vi "main test.vi"() -> ()   [LabVIEW 2023, in "Thermotron 8800.lvlib"]
uses:
  Thermotron 8800.lvlib
  Private/AuxSelection.ctl
  Private/ActiveChannels.ctl
  Private/Live Aux Number.ctl
  Private/group.ctl
  Private/control module number.ctl
  Private/AnalogInputChannelNumber.ctl
  Private/ThermAlarmNumberBase0.ctl
  Private/get set.ctl
  Private/AnalogInputChannelNumber 1-4.ctl
  Private/Enabled Off On.ctl
  Private/Power Recovery Mode.ctl
  Private/OptionWordSelection.ctl
  Private/ThermAlarmNumber.ctl
  Private/Celcius or Fahrenheit.ctl
  Private/reset.ctl
  <vilib>/NI/Progress Bar/Controls/Update Bar Actions.ctl
panel:
  in  "Input parms":T1={"Controlled stop mode (1=enable; 0=disable)"=1, "Controlled stop set point (0 - 50 deg C)"=30, "Controlled stop purge time (0-3600 seconds)"=10, "Controlled stop deviation (0 - 999.9 deg C)"=5.2, "Controlled stop control mode (1=on; 0=off)"=1}
  out "Software version":string
  out "Temperature scale text":string
  out "Temperature scale\n(0=Celcius; 1=Fahrenheit)":u8
  out "Temperature scale":string
  out "Temperature scale result":string
  out "Time left string 3":string
  out "Time left string 2":string
  out "seconds":i32
  out "minutes":i32
  out "hours":i32
  out "Time left cluster":T2
  out "Time left string 4":string
  out "Time left string 1":string
  out "Throttle reading":i8 format="%0.1f"
  out "Throttle reading string":string
  out "ThermAlarm temperature":i32
  out "ThermAlarm temperature string":string
  out "ThermAlarm analog input value":i32
  out "ThermAlarm analog input value string":string
  out "Reset watchdog timer result":string
  out "Manual ramp setting":sgl
  out "Manual ramp setting string":string
  out "Manual ramp setting status":string
  out "Monitor channel value":sgl
  out "Monitor Channel Value String":string
  out "Operating mode binary":string
  out "Operating mode":u8
  out "Operating mode string":string
  out "Service request event mask binary":string
  out "Service request event mask":i32
  out "Controlled stop parms response":string
  out "Controlled stop parms response from set":string
  out "Number of loops string":string
  out "Number of loops":i32
  out "Next interval":i32
  out "Option response get":string
  out "Option response set":string
  out "High process alarm limit":string
  out "Low process alarm limit":string
  out "Parm response 2":string
  out "Parm response":string
  out "Parameter values response":string
  out "Currently loaded program name response":string
  out "Parameter group":string
  out "Parameter group response":string
  out "8800 program":string
  out "8800 response":string
  out "Program time":string
  out "Program time remaining":string
  out "Process Variable":string
  out "Power fail recovery response":string
  out "Power fail recovery set response":string
  out "Refrigeration system status binary string":string
  out "Refrigeration system status":i32
  out "Refrigeration system status string":string
  out "Refrig system pressures":string
  out "Resume result":string
  out "Real time clock":string
  out "Real time clock set result":string
  out "Stop code":string
  out "reset screen response":string
  out "Chamber serial number":string
  out "Setpoint":dbl format="%.1f"
  out "Setpoint status":string
  out "Service request event mask status":string
  out "Service request event mask string":string
  out "Service request binary string":string
  out "Service request status":i32
  out "Service request status string":string
  out "Service request interval":string
  out "Service request interval status":string
  out "Access level response set":string
  out "Access level response get":string
  out "Loops left?":string
  out "Loops left status":string
  out "Light Status from Set":string
  out "Light Status from Get":string
  out "Enabled? (0=disabled, 1=enabled) 2":i32
  out "Live Aux State (0=off, 1=on) 2":i32
  out "Enabled? (0=disabled, 1=enabled)":i32
  out "Live Aux State (0=off, 1=on)":i32
  in  "State (o=off, 1=on)":i8=1 min=0 max=1 step=1
  in  "Live Aux Number (1-8)":T3=2 min=1 max=8
  out "Language Mode Integer":i32
  out "Language Mode string":string
  out "Current interval initial value":sgl
  out "Current interval initial value string":string
  out "Interval Time":string
  out "analog input channel available?":i32
  in  "Aux Cluster 2":T5={"Group 1 Aux box input"=[2, 4, 5], "Group 2 Aux box input"=[5, 7], "Group 1 Aux code input"=0, "Group 2 Aux code input"=0, "Aux selector box"=TRUE} {"Group 2 Aux code input" min=0 max=255 step=1; "Group 1 Aux code input" min=0 max=255 step=1}
  in  "Interval Parameters Cluster 2":T6={"Final Value 1"=33.2, "Final Value 2"=43.7, "Final Value 3"=0.0, "Final Value 4"=0.0, "Deviation 1"=4.0, "Deviation 2"=5.0, "Deviation 3"=0.0, "Deviation 4"=0.0, "hours"=3, "minutes"=6, "seconds"=7, "Parameter Group"=3, "Number Of Loops"=4, "Next Interval"=1} {"Next Interval" min=0 max=300 step=1; "Number Of Loops" min=0 max=9999 step=1; "Parameter Group" min=1 max=4 step=1; "seconds" min=0 max=99 step=1; "minutes" min=0 max=99 step=1; "hours" min=0 max=99 step=1}
  in  "Interval Parameters Cluster 1":T6={"Final Value 1"=31.2, "Final Value 2"=41.7, "Final Value 3"=0.0, "Final Value 4"=0.0, "Deviation 1"=3.3, "Deviation 2"=4.4, "Deviation 3"=0.0, "Deviation 4"=0.0, "hours"=2, "minutes"=4, "seconds"=5, "Parameter Group"=2, "Number Of Loops"=0, "Next Interval"=2} {"Next Interval" min=0 max=300 step=1; "Number Of Loops" min=0 max=9999 step=1; "Parameter Group" min=1 max=4 step=1; "seconds" min=0 max=99 step=1; "minutes" min=0 max=99 step=1; "hours" min=0 max=99 step=1}
  out "8800 Get Response INTV2":string
  out "Program number of intervals from set":string
  out "Program get number of intervals":string
  out "8800 Get Response from INTV 0":string
  out "8800 Set Response from INTV 0":string
  in  "Interval Parameters Cluster 0":T6={"Final Value 1"=29.2, "Final Value 2"=39.7, "Final Value 3"=0.0, "Final Value 4"=0.0, "Deviation 1"=1.1, "Deviation 2"=2.2, "Deviation 3"=0.0, "Deviation 4"=0.0, "hours"=1, "minutes"=2, "seconds"=3, "Parameter Group"=1, "Number Of Loops"=0, "Next Interval"=1} {"Next Interval" min=0 max=300 step=1; "Number Of Loops" min=0 max=9999 step=1; "Parameter Group" min=1 max=4 step=1; "seconds" min=0 max=99 step=1; "minutes" min=0 max=99 step=1; "hours" min=0 max=99 step=1}
  in  "Active Channels Cluster":T8={"Active Channels box input"=[1, 2], "Active Channels code input"=7, "Active Channels selector T(box) F(code)"=FALSE} {"Active Channels code input" min=0 max=15 step=1}
  in  "Aux Cluster 1":T5={"Group 1 Aux box input"=[1, 3], "Group 2 Aux box input"=[6, 8], "Group 1 Aux code input"=9, "Group 2 Aux code input"=12, "Aux selector box"=FALSE} {"Group 2 Aux code input" min=0 max=255 step=1; "Group 1 Aux code input" min=0 max=255 step=1}
  out "8800 Get Response from INTV1":string
  out "8800 Set Response from INTV 2":string
  out "8800 Set Response from INTV1":string
  out "Interval Number":i32
  out "Interval Number string":string
  out "Last error code":string
  out "8800 Response Identification scpi":string
  out "8800 Response Identification":string
  out "8800 Response":string
  out "Data Type":string
  out "Reference Data Type":string
  out "Door Status":string
  out "Program Directory":string
  out "Digital Output Status binary extended":string
  out "Digital Output Status extended":i32
  out "Digital Output Status string extended":string
  out "Digital Output Status binary":string
  out "Digital Output Status":i32
  out "Digital Output Status string":string
  out "Digital Input Status binary":string
  out "Digital Input Status":i32
  out "Digital Input Status string":string
  out "set deviation response":string
  out "get deviation response":string
  out "Active channel status":i32
  out "Active channel status string":string
  out "version number of control module":string
  out "Channel on and configured status binary":string
  out "analog therm-alarm settings":string[](array[string])
  out "set result talrm settings":string
  out "Configured Options binary string":string
  out "Configured Options":i32
  out "Configured Options string":string
  out "Name of channel":string
  out "Comm status String Value":string
  out "Comm status Value":i32
  out "Channel on and configured status":string
  out "channel run time":string
  out "channel configuration information":string
  out "ascii units character":string
  out "Alarm status":i32
  out "Aux Decimal Value":i32
  out "Aux String Value":string
  out "Alarm status string":string
  out "ThermAlarm analog input units value":string
  out "Instrument Firmware Revision":string
  out "Instrument Driver Revision":string
  out "error out":errorcluster
  in  "error in (no error)":errorcluster
  in  "VISA resource name":refnum<visa-resource-name>="TCPIP::192.168.2.102::8888::SOCKET"
  # "Select Aux boxes"
  # "Select Aux code"
  # "Select Active Channels boxes"
  # "Select Active Channels code"
  # "Select Aux boxes"
  # "Select Aux code"
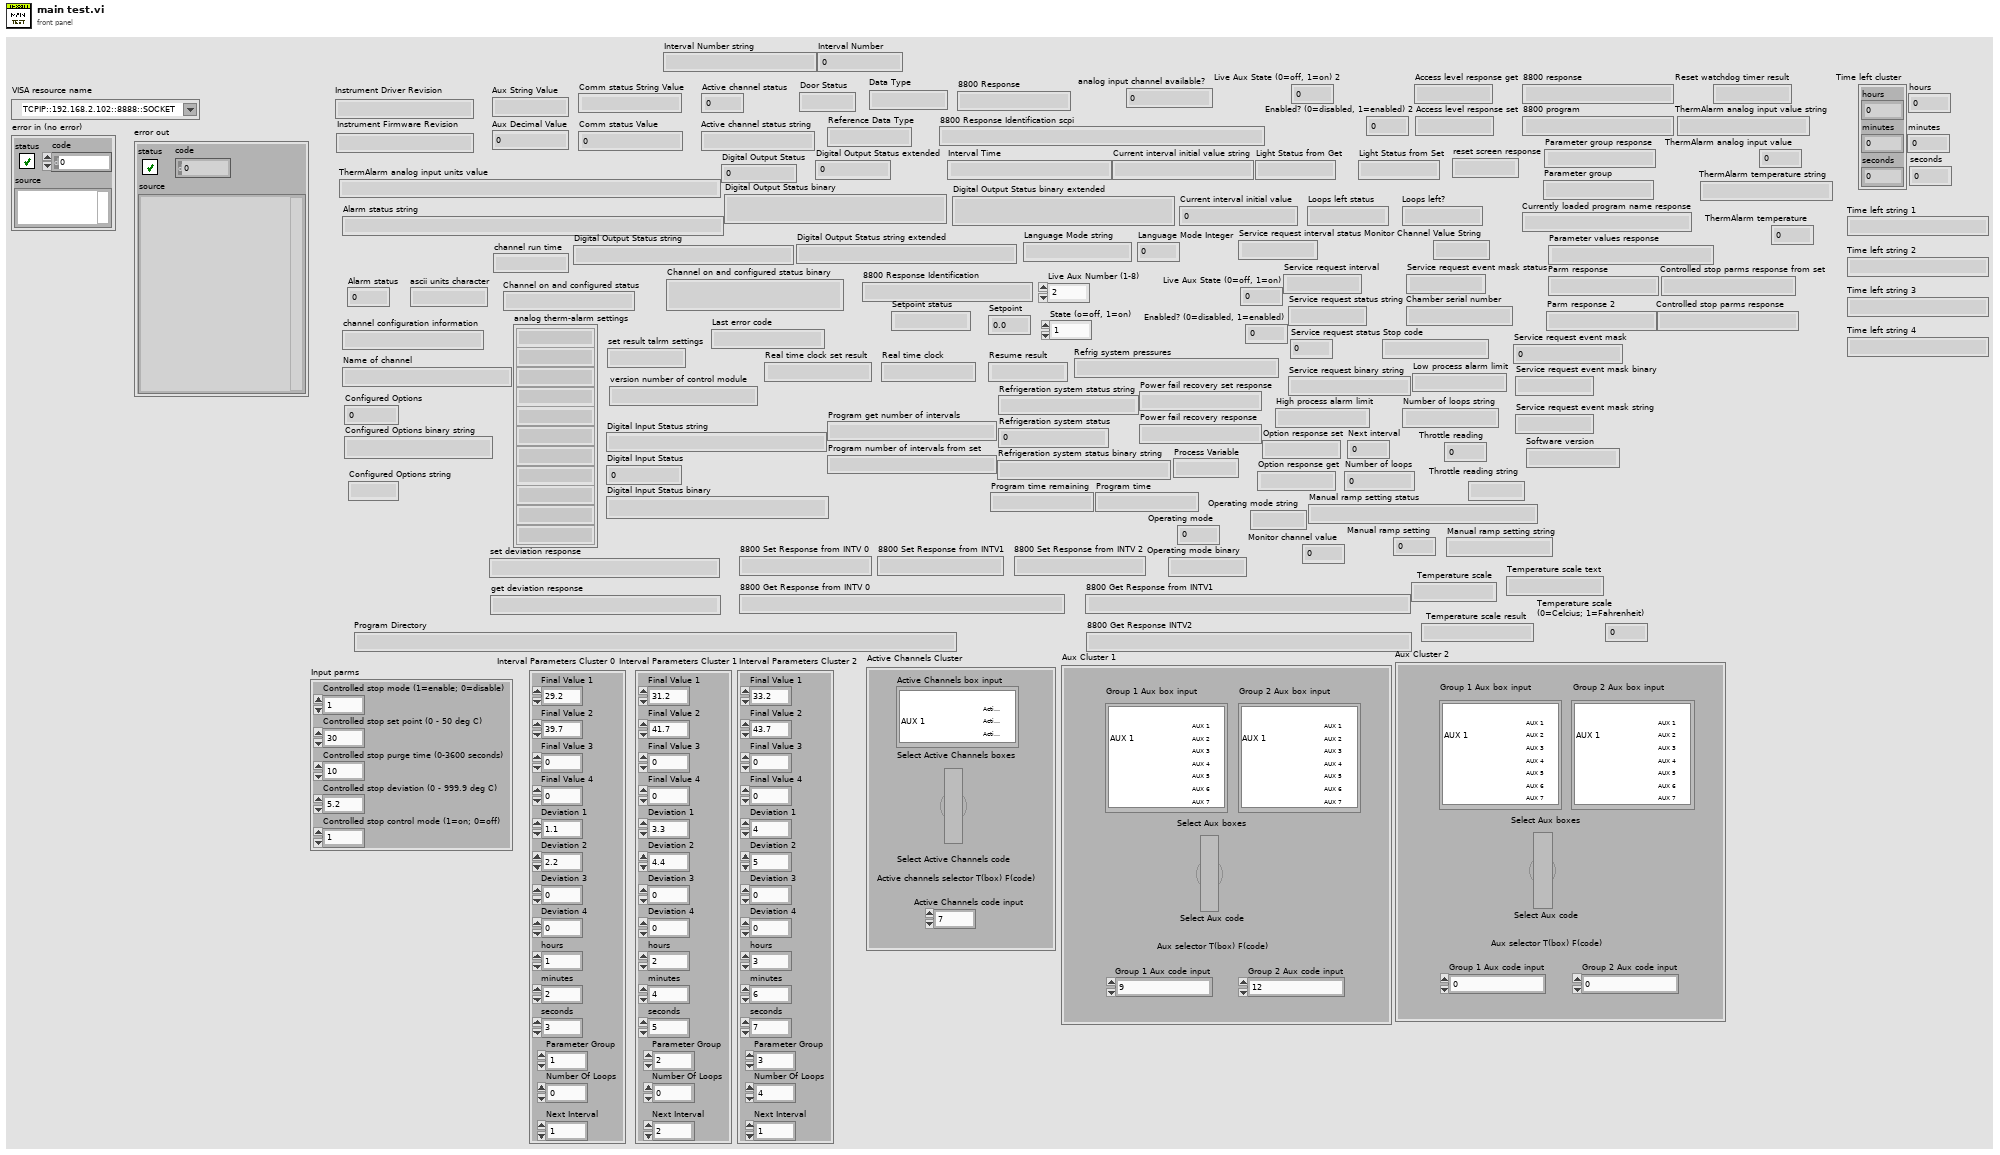
[diagram p1: front panel]
types:
  T1 = cluster{"Controlled stop mode (1=enable; 0=disable)":u8, "Controlled stop set point (0 - 50 deg C)":u8, "Controlled stop purge time (0-3600 seconds)":u16, "Controlled stop deviation (0 - 999.9 deg C)":sgl, "Controlled stop control mode (1=on; 0=off)":u8}
  T2 = cluster{"hours":i32, "minutes":i32, "seconds":i32}
  T3 = typedef "Thermotron 8800.lvlib/Live Aux Number.ctl" = i8
  T4 = typedef "Thermotron 8800.lvlib/AuxSelection.ctl" = i32[]
  T5 = cluster{"Group 1 Aux box input":T4, "Group 2 Aux box input":T4, "Group 1 Aux code input":i32, "Group 2 Aux code input":i32, "Aux selector box":bool}
  T6 = cluster{"Final Value 1":sgl, "Final Value 2":sgl, "Final Value 3":sgl, "Final Value 4":sgl, "Deviation 1":sgl, "Deviation 2":sgl, "Deviation 3":sgl, "Deviation 4":sgl, "hours":i8, "minutes":i8, "seconds":i8, "Parameter Group":i8, "Number Of Loops":i16, "Next Interval":i16}
  T7 = typedef "Thermotron 8800.lvlib/ActiveChannels.ctl" = i32[]
  T8 = cluster{"Active Channels box input":T7, "Active Channels code input":i32, "Active Channels selector T(box) F(code)":bool}
  T9 = cluster{"Hours\n(0-99)":u8, "Minutes\n(0-5999)":u16, "Seconds\n(0-359999)":u32}
  T10 = typedef "Thermotron 8800.lvlib/reset.ctl" = u16
  T11 = cluster{"warn":i32, "mute":i32, "High Limit":i32, "Low Limit":i32, "delay":i32, "reset":T10}
  T12 = cluster{"Month":string, "Day":string, "Hour":string, "Minute":string}
  T13 = typedef "Thermotron 8800.lvlib/Celcius or Fahrenheit.ctl" = u8
  T14 = typedef "Thermotron 8800.lvlib/get set.ctl" = enum16{"get", "set"}
  T15 = typedef "Thermotron 8800.lvlib/AnalogInputChannelNumber.ctl" = u16
  T16 = typedef "Thermotron 8800.lvlib/ThermAlarmNumber.ctl" = u16
  T17 = typedef "Thermotron 8800.lvlib/AnalogInputChannelNumber 1-4.ctl" = u16
  T18 = typedef "Thermotron 8800.lvlib/OptionWordSelection.ctl" = u16
  T19 = cluster{"Heat Gain":sgl, "Heat IT":u16, "Heat Off":sgl, "Cool Off":sgl, "Cool Gain":sgl, "Cool IT":u16}
  T20 = cluster{"Heat PB":sgl, "Heat IT":u16, "Heat TL":sgl, "Cool TL":sgl, "Cool PB":sgl, "Cool IT":u16}
  T21 = typedef "Thermotron 8800.lvlib/Power Recovery Mode.ctl" = u8
  T22 = typedef "Thermotron 8800.lvlib/Enabled Off On.ctl" = u8
  T23 = typedef "Thermotron 8800.lvlib/control module number.ctl" = u16
  T24 = typedef "Thermotron 8800.lvlib/ThermAlarmNumberBase0.ctl" = u16
  T25 = typedef "Thermotron 8800.lvlib/group.ctl" = enum16{"Group1", "Group2"}
  T26 = typedef "Progress Bar.lvlib/Update Bar Actions.ctl" = enum16{"Add To Existing", "Set to Value"}
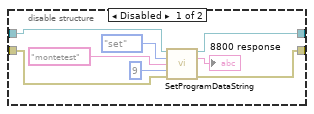
[diagram p2: hidden frame]
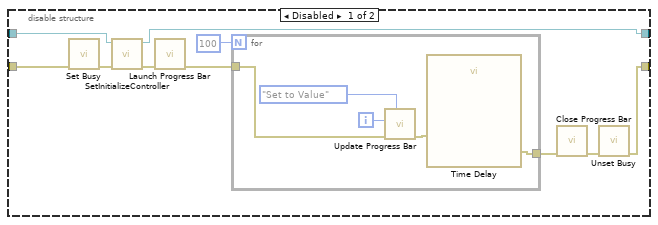
[diagram p3: hidden frame]
diagram:
  w17 = T13 0 items=["Celcius", "Fahrenheit"] ("Temperature scale")
  w24 = get_set."get" ("get/set")
  w43 = get_set."set" ("get/set")
  w50 = T15 2 items=["Channel 1"=1, "Channel 2"=2, "Channel 3"=3, "Channel 4"=4, "Channel 5"=5, "Channel 6"=6, "Channel 7"=7, "Channel 8"=8] ("Channel Number (1-8)")
  w55 = T16 1 items=["ThermAlarm 1"=1, "ThermAlarm 2"=2, "ThermAlarm 3"=3, "ThermAlarm 4"=4] ("ThermAlarm number")
  w71 = T17 1 items=["Channel 1"=1, "Channel 2"=2, "Channel 3"=3, "Channel 4"=4] ("Channel Number (1-4)")
  w106 = T18 8 items=["Product temperature control"=1, "Humidity system"=2, "Low humidity system"=4, "GSoak"=8, "Purge"=16, "Cascade refrigeration"=32, "Power Save mode"=64, "Single-stage refrig."=128, "Altitude"=512, "Mechanical boost"=1024, "Product dewpoint control"=32768] ("Option (may be added for multiple)")
  w116 = T17 1 items=["Channel 1"=1, "Channel 2"=2, "Channel 3"=3, "Channel 4"=4] ("Channel Number (1-4)")
  w141 = "%.1f" ("format string")
  w148 = string[] [","] ("delimiters (\\s,\\t,\\r,\\n)")
  w133 = u8 1 ("Parameter group number (1-4)")
  w134 = T17 1 items=["Channel 1"=1, "Channel 2"=2, "Channel 3"=3, "Channel 4"=4] ("Control channel number (1-4)")
  w135 = get_set."set" ("get/set")
  w195 = T21 2 items=["stop", "hold", "run", "restart"] ("Power Recovery Mode")
  w199 = T22 1 items=["Off", "On"] ("Enabled?")
  w209 = T17 1 items=["Channel 1"=1, "Channel 2"=2, "Channel 3"=3, "Channel 4"=4] ("Refrigeration system number (1-4)")
  w211 = T17 1 items=["Channel 1"=1, "Channel 2"=2, "Channel 3"=3, "Channel 4"=4] ("Refrig system number (1-4)")
  w235 = T17 1 items=["Channel 1"=1, "Channel 2"=2, "Channel 3"=3, "Channel 4"=4] ("Channel Number (1-4)")
  w290 = get_set."get" ("get/set")
  w291 = get_set."set" ("get/set")
  w319 = T17 1 items=["Channel 1"=1, "Channel 2"=2, "Channel 3"=3, "Channel 4"=4] ("Channel Number (1-4)")
  w326 = T16 1 items=["ThermAlarm 1"=1, "ThermAlarm 2"=2, "ThermAlarm 3"=3, "ThermAlarm 4"=4] ("ThermAlarm number")
  w354 = "test" ("8800 Program Name")
  w365 = i16 0 ("Interval Number")
  w338 = i16 2 ("Interval Number")
  w360 = i16 1 ("Interval Number")
  w337 = get_set."get" ("get/set")
  w366 = get_set."set" ("get/set")
  w370 = u16 32 items=["Product temperature control"=1, "Humidity system"=2, "Low humidity system"=4, "GSoak"=8, "Purge"=16, "Cascade refrigeration"=32, "Power Save mode"=64, "Single-stage refrigeration"=128, "Altitude"=512, "Mechanical boost"=1024, "Product dew point control"=32768] ("Options")
  w333 = u16 32 items=["Product temperature control"=1, "Humidity system"=2, "Low humidity system"=4, "GSoak"=8, "Purge"=16, "Cascade refrigeration"=32, "Power Save mode"=64, "Single-stage refrigeration"=128, "Altitude"=512, "Mechanical boost"=1024, "Product dew point control"=32768] ("Options")
  w369 = u16 2 items=["Product temperature control"=1, "Humidity system"=2, "Low humidity system"=4, "GSoak"=8, "Purge"=16, "Cascade refrigeration"=32, "Power Save mode"=64, "Single-stage refrigeration"=128, "Altitude"=512, "Mechanical boost"=1024, "Product dew point control"=32768] ("Options")
  w332 = u16 1024 items=["Product temperature control"=1, "Humidity system"=2, "Low humidity system"=4, "GSoak"=8, "Purge"=16, "Cascade refrigeration"=32, "Power Save mode"=64, "Single-stage refrigeration"=128, "Altitude"=512, "Mechanical boost"=1024, "Product dew point control"=32768] ("Options")
  w331 = u16 2 items=["Product temperature control"=1, "Humidity system"=2, "Low humidity system"=4, "GSoak"=8, "Purge"=16, "Cascade refrigeration"=32, "Power Save mode"=64, "Single-stage refrigeration"=128, "Altitude"=512, "Mechanical boost"=1024, "Product dew point control"=32768] ("Options")
  w393 = T17 1 items=["Channel 1"=1, "Channel 2"=2, "Channel 3"=3, "Channel 4"=4] ("Channel Number (1-4)")
  w417 = T23 2 items=["control module 1"=1, "control module 2"=2, "control module 3"=3, "control module 4"=4] ("control module number")
  w430 = T17 1 items=["Channel 1"=1, "Channel 2"=2, "Channel 3"=3, "Channel 4"=4] ("Channel Number (1-4)")
  w442 = T24 0 items=["ThermAlarm 1", "ThermAlarm 2", "ThermAlarm 3", "ThermAlarm 4"] ("ThermAlarm number")
  w446 = T15 1 items=["Channel 1"=1, "Channel 2"=2, "Channel 3"=3, "Channel 4"=4, "Channel 5"=5, "Channel 6"=6, "Channel 7"=7, "Channel 8"=8] ("Channel Number")
  w444 = T15 2 items=["Channel 1"=1, "Channel 2"=2, "Channel 3"=3, "Channel 4"=4, "Channel 5"=5, "Channel 6"=6, "Channel 7"=7, "Channel 8"=8] ("Channel Number")
  w445 = T15 1 items=["Channel 1"=1, "Channel 2"=2, "Channel 3"=3, "Channel 4"=4, "Channel 5"=5, "Channel 6"=6, "Channel 7"=7, "Channel 8"=8] ("Channel Number")
  w448 = T23 1 items=["control module 1"=1, "control module 2"=2, "control module 3"=3, "control module 4"=4] ("control module number")
  w456 = T16 1 items=["ThermAlarm 1"=1, "ThermAlarm 2"=2, "ThermAlarm 3"=3, "ThermAlarm 4"=4, "ThermAlarm 5"=5, "ThermAlarm 6"=6, "ThermAlarm 7"=7, "ThermAlarm 8"=8] ("ThermAlarm number")
  # "note: SRQM and SRQB are already done"
  # "main test.vi"
  n1 = call "Initialize.vi"("error in (no error)"="error in (no error)", "VISA resource name"="VISA resource name") -> ("error out"=w513:errorcluster, "VISA resource name out"=w512:refnum<visa-resource-name>)  [unwired: 7 in, 1 out]
  n2 = call "Reset.vi"("error in (no error)"=w513, "VISA resource name"=w512) -> ("error out"=w489:errorcluster, "VISA resource name out"=w490:refnum<visa-resource-name>)  [unwired: 8 in]
  n3 = call "Revision Query.vi"("error in (no error)"=w489, "VISA resource name"=w490) -> ("error out"=w508:errorcluster, "Instrument Firmware Revision"=→"Instrument Firmware Revision":string, "Instrument Driver Revision"=→"Instrument Driver Revision":string, "VISA resource name out"=w509:refnum<visa-resource-name>)  [unwired: 6 in]
  n4 = call "GetThermAlarmAnalogInputUnitsValue.vi"("error in"=w508, "ThermAlarm number"=w456, "VISA resource name"=w509) -> ("error out"=w506:errorcluster, "ThermAlarm analog input units value"=→"ThermAlarm analog input units value":string, "VISA resource name out"=w505:refnum<visa-resource-name>)  [unwired: 6 in]
  n5 = call "GetAlarmStatus.vi"("error in"=w506, "Channel Number"=w446, "VISA resource name"=w505) -> ("error out"=w496:errorcluster, "Alarm status"=→"Alarm status":i32, "Alarm status string"=→"Alarm status string":string, "VISA resource name out"=w493:refnum<visa-resource-name>)  [unwired: 5 in]
  n6 = call "GetSetAux.vi"("Aux code input"=173, "error in"=w496, "Group"=group."Group1", "get/set"=get_set."set", "VISA resource name"=w493) -> ("error out"=w495:errorcluster, "VISA resource name out"=w492:refnum<visa-resource-name>)  [unwired: 3 in, 2 out]
  n7 = call "SetRunManual.vi"("error in"=w495, "VISA resource name"=w492) -> ("error out"=w494:errorcluster, "VISA resource name out"=w491:refnum<visa-resource-name>)  [unwired: 7 in, 1 out]
  n8 = call "GetSetAux.vi"("error in"=w494, "Group"=group."Group1", "get/set"=get_set."get", "VISA resource name"=w491) -> ("error out"=w484:errorcluster, "Aux Decimal Value"=→"Aux Decimal Value":i32, "Aux String Value"=→"Aux String Value":string, "VISA resource name out"=w485:refnum<visa-resource-name>)  [unwired: 4 in]
  n9 = call "GetPVUnitsChar.vi"("error in"=w484, "Channel number"=1, "VISA resource name"=w485) -> ("error out"=w482:errorcluster, "ascii units character"=→"ascii units character":string, "VISA resource name out"=w483:refnum<visa-resource-name>)  [unwired: 6 in]
  n10 = call "GetProcessChanConfig.vi"("error in"=w482, "Channel Number"=w445, "VISA resource name"=w483) -> ("error out"=w480:errorcluster, "channel configuration information"=→"channel configuration information":string, "VISA resource name out"=w479:refnum<visa-resource-name>)  [unwired: 6 in]
  n11 = call "GetChanRunTime.vi"("error in"=w480, "Channel Number"=w444, "VISA resource name"=w479) -> ("error out"=w477:errorcluster, "channel run time"=→"channel run time":string, "VISA resource name out"=w476:refnum<visa-resource-name>)  [unwired: 6 in]
  n12 = call "GetChanOnAndConfigStatus.vi"("error in"=w477, "VISA resource name"=w476) -> ("error out"=w472:errorcluster, "Channel on and configured status binary"=→"Channel on and configured status binary":string, "Channel on and configured status string"=→"Channel on and configured status":string, "VISA resource name out"=w470:refnum<visa-resource-name>)  [unwired: 6 in]
  n13 = call "GetSetCommStatus.vi"("error in"=w472, "Coded integer comm status"=1, "get/set"=get_set."set", "VISA resource name"=w470) -> ("error out"=w471:errorcluster, "VISA resource name out"=w469:refnum<visa-resource-name>)  [unwired: 4 in, 2 out]
  n14 = call "GetSetCommStatus.vi"("error in"=w471, "get/set"=get_set."get", "VISA resource name"=w469) -> ("error out"=w466:errorcluster, "Comm status Value"=→"Comm status Value":i32, "Comm status String Value"=→"Comm status String Value":string, "VISA resource name out"=w467:refnum<visa-resource-name>)  [unwired: 5 in]
  n15 = call "GetChanName.vi"("error in"=w466, "Channel number"=1, "VISA resource name"=w467) -> ("error out"=w463:errorcluster, "Name of channel"=→"Name of channel":string, "VISA resource name out"=w462:refnum<visa-resource-name>)  [unwired: 6 in]
  n16 = call "GetConfiguredOptions.vi"("VISA resource name"=w462, "error in"=w463) -> ("VISA resource name out"=w453:refnum<visa-resource-name>, "Configured Options string"=→"Configured Options string":string, "Configured Options"=→"Configured Options":i32, "Configured Options binary string"=→"Configured Options binary string":string, "error out"=w454:errorcluster)  [unwired: 9 in]
  n17 = call "GetSetThermAlarmSettings.vi"("VISA resource name"=w453, "ThermAlarm number"=w442, "get/set"=get_set."set", "Input cluster"=T11 {"warn"=3, "mute"=99, "High Limit"=6, "Low Limit"=2, "delay"=4, "reset"=1}, "error in"=w454) -> ("VISA resource name out"=w452:refnum<visa-resource-name>, "set response"=→"set result talrm settings":string, "error out"=w451:errorcluster)  [unwired: 10 in, 2 out]
  n18 = call "GetSetThermAlarmSettings.vi"("VISA resource name"=w452, "ThermAlarm number"=w442, "get/set"=get_set."get", "error in"=w451) -> ("VISA resource name out"=w449:refnum<visa-resource-name>, "get response"=→"analog therm-alarm settings":string[], "error out"=w450:errorcluster)  [unwired: 11 in, 2 out]
  n19 = call "GetControlModuleVersion.vi"("error in"=w450, "control module number"=w448, "VISA resource name"=w449) -> ("error out"=w440:errorcluster, "version number of control module"=→"version number of control module":string, "VISA resource name out"=w439:refnum<visa-resource-name>)  [unwired: 6 in]
  n20 = call "GetActiveChannelStatus.vi"("error in"=w440, "VISA resource name"=w439) -> ("error out"=w436:errorcluster, "Active channel status"=→"Active channel status":i32, "Active channel status string"=→"Active channel status string":string, "VISA resource name out"=w435:refnum<visa-resource-name>)  [unwired: 6 in]
  n21 = call "GetSetDeviation.vi"("Deviation value"=21.1, "error in"=w436, "Channel Number (1-4)"=w430, "get/set"=get_set."set", "VISA resource name"=w435) -> ("error out"=w434:errorcluster, "Deviation"=→"set deviation response":string, "VISA resource name out"=w433:refnum<visa-resource-name>)  [unwired: 4 in]
  n22 = call "GetSetDeviation.vi"("error in"=w434, "Channel Number (1-4)"=w430, "get/set"=get_set."get", "VISA resource name"=w433) -> ("error out"=w425:errorcluster, "Deviation"=→"get deviation response":string, "VISA resource name out"=w426:refnum<visa-resource-name>)  [unwired: 5 in]
  n23 = call "GetDigitalInputStatus.vi"("VISA resource name"=w426, "error in"=w425) -> ("VISA resource name out"=w418:refnum<visa-resource-name>, "Digital Input Status string"=→"Digital Input Status string":string, "Digital Input Status"=→"Digital Input Status":i32, "Digital Input Status binary"=→"Digital Input Status binary":string, "error out"=w419:errorcluster)  [unwired: 9 in]
  n24 = call "GetDigitalOutputStatus.vi"("VISA resource name"=w418, "error in"=w419) -> ("VISA resource name out"=w421:refnum<visa-resource-name>, "Digital Output Status string"=→"Digital Output Status string":string, "Digital Output Status"=→"Digital Output Status":i32, "Digital Output Status binary"=→"Digital Output Status binary":string, "error out"=w420:errorcluster)  [unwired: 9 in]
  n25 = call "GetDigitalOutputStatus.vi"("VISA resource name"=w421, "control module number"=w417, "Extended?"=TRUE, "error in"=w420) -> ("VISA resource name out"=w406:refnum<visa-resource-name>, "Digital Output Status string"=→"Digital Output Status string extended":string, "Digital Output Status"=→"Digital Output Status extended":i32, "Digital Output Status binary"=→"Digital Output Status binary extended":string, "error out"=w407:errorcluster)  [unwired: 7 in]
  n26 = call "GetProgramDirectory.vi"("error in"=w407, "PathName"="\\", "VISA resource name"=w406) -> ("error out"=w403:errorcluster, "Program Directory"=→"Program Directory":string, "VISA resource name out"=w402:refnum<visa-resource-name>)  [unwired: 6 in]
  n27 = call "GetDoorStatus.vi"("error in"=w403, "VISA resource name"=w402) -> ("error out"=w400:errorcluster, "Door Status"=→"Door Status":string, "VISA resource name out"=w399:refnum<visa-resource-name>)  [unwired: 7 in]
  n28 = call "GetReferenceDataType.vi"("error in"=w400, "Channel Number"=1, "VISA resource name"=w399) -> ("error out"=w397:errorcluster, "Reference Data Type"=→"Reference Data Type":string, "VISA resource name out"=w396:refnum<visa-resource-name>)  [unwired: 6 in]
  n29 = call "GetDataType.vi"("error in (no error)"=w397, "Channel Number (1-4)"=w393, "VISA resource name"=w396) -> ("error out"=w392:errorcluster, "Data Type"=→"Data Type":string, "VISA resource name out"=w391:refnum<visa-resource-name>)  [unwired: 6 in]
  n30 = call "SetHold.vi"("error in"=w392, "VISA resource name"=w391) -> ("error out"=w388:errorcluster, "8800 Response"=→"8800 Response":string, "VISA resource name out"=w389:refnum<visa-resource-name>)  [unwired: 7 in]
  n31 = call "GetDeviceIdentification.vi"("error in"=w388, "VISA resource name"=w389) -> ("error out"=w386:errorcluster, "8800 Response Identification"=→"8800 Response Identification":string, "VISA resource name out"=w385:refnum<visa-resource-name>)  [unwired: 7 in]
  n32 = call "GetDeviceIdentificationSCPI.vi"("error in"=w386, "VISA resource name"=w385) -> ("error out"=w383:errorcluster, "8800 Response Identification"=→"8800 Response Identification scpi":string, "VISA resource name out"=w382:refnum<visa-resource-name>)  [unwired: 7 in]
  n33 = call "GetLastErrorCode.vi"("error in"=w383, "VISA resource name"=w382) -> ("error out"=w376:errorcluster, "Last error code"=→"Last error code":string, "VISA resource name out"=w380:refnum<visa-resource-name>)  [unwired: 7 in]
  n34 = disable-structure shown="Enabled" {
    disable-tunnel: w380 -> [w526 w533]
    disable-tunnel: [w525 w533] -> w379
    disable-tunnel: w376 -> [w524 w532]
    disable-tunnel: [w522 w532] -> w375
    frame Disabled {
      n35 = call <vilib>:"Set Busy.vi"("error in (no error)"=w524) -> ("error out"=w523:errorcluster)  [unwired: 9 in, 1 out]
      n36 = call <instrlib>:"SetInitializeController.vi"("error in"=w523, "VISA resource name"=w526) -> ("error out"=w521:errorcluster, "VISA resource name out"=w525:refnum<visa-resource-name>)  [unwired: 8 in]
      n37 = call <vilib>:"Launch Progress Bar.vi"("error in (no error)"=w521) -> ("error out"=w520:errorcluster)  [unwired: 9 in, 1 out]
      n38 = for {
        N: 100 -> [_]
        tunnel: w520 -> [w531]
        tunnel: [w529] -> w519
        i -> [w527]
        n39 = call <vilib>:"Update Progress Bar.vi"("Action"=Update_Bar_Actions."Set to Value", "error in (no error)"=w531, "Value"=w527) -> ("error out"=w530:errorcluster)  [unwired: 8 in]
        n40 = call "Time Delay"("error in (no error)"=w530) -> ("error out"=w529:errorcluster)  [unwired: 10 in]
      }
      n41 = call <vilib>:"Close Progress Bar.vi"("error in (no error)"=w519) -> ("error out"=w518:errorcluster)  [unwired: 9 in, 1 out]
      n42 = call <vilib>:"Unset Busy.vi"("error in (no error)"=w518) -> ("error out"=w522:errorcluster)  [unwired: 10 in]
    }
    frame Enabled {
    }
  }
  n43 = call "GetIntervalNumber.vi"("error in"=w375, "VISA resource name"=w379) -> ("error out"=w359:errorcluster, "Interval Number"=→"Interval Number":i32, "Interval Number string"=→"Interval Number string":string, "VISA resource name out"=w358:refnum<visa-resource-name>)  [unwired: 6 in]
  n44 = call "GetSetProgramDataString.vi"("VISA resource name"=w358, "get/set"=get_set."set", "8800 Program Name"=w354, "Number of Intervals"=i16 2, "error in"=w359) -> ("VISA resource name out"=w351:refnum<visa-resource-name>, "Program get number of intervals"=→"Program number of intervals from set":string, "error out"=w352:errorcluster)  [unwired: 8 in]
  n45 = call "GetSetProgramIntervalString.vi"("VISA resource name"=w351, "get/set"=w366, "Interval Number (Interval 0 is special case)"=w365, "Interval Parameters Cluster\n(only first four values are\nused for Interval 0)"="Interval Parameters Cluster 0", "error in"=w352, "Active Channels Cluster ( only used for Interval 0)"="Active Channels Cluster") -> ("VISA resource name out"=w348:refnum<visa-resource-name>, "8800 Response"=→"8800 Set Response from INTV 0":string, "error out"=w349:errorcluster)  [unwired: 11 in]
  n46 = Compound Arithmetic op=unknown(w369, w333, w370) -> (w362:u16)
  n47 = Compound Arithmetic op=unknown(w331, w332, w333) -> (w330:u16)
  n48 = call "GetSetProgramIntervalString.vi"("VISA resource name"=w348, "get/set"=w366, "Interval Number (Interval 0 is special case)"=w360, "Aux Cluster"="Aux Cluster 1", "Interval Parameters Cluster\n(only first four values are\nused for Interval 0)"="Interval Parameters Cluster 1", "error in"=w349, "Options"=w362) -> ("VISA resource name out"=w372:refnum<visa-resource-name>, "8800 Response"=→"8800 Set Response from INTV1":string, "error out"=w373:errorcluster)  [unwired: 10 in]
  n49 = call "GetSetProgramIntervalString.vi"("VISA resource name"=w372, "get/set"=w366, "Interval Number (Interval 0 is special case)"=w338, "Aux Cluster"="Aux Cluster 2", "Interval Parameters Cluster\n(only first four values are\nused for Interval 0)"="Interval Parameters Cluster 2", "error in"=w373, "Options"=w330) -> ("VISA resource name out"=w346:refnum<visa-resource-name>, "8800 Response"=→"8800 Set Response from INTV 2":string, "error out"=w347:errorcluster)  [unwired: 10 in]
  n50 = call "GetSetProgramIntervalString.vi"("VISA resource name"=w346, "get/set"=w337, "Interval Number (Interval 0 is special case)"=w365, "error in"=w347) -> ("VISA resource name out"=w345:refnum<visa-resource-name>, "8800 Response"=→"8800 Get Response from INTV 0":string, "error out"=w344:errorcluster)  [unwired: 13 in]
  n51 = call "GetSetProgramIntervalString.vi"("VISA resource name"=w345, "get/set"=w337, "Interval Number (Interval 0 is special case)"=w360, "error in"=w344) -> ("VISA resource name out"=w340:refnum<visa-resource-name>, "8800 Response"=→"8800 Get Response from INTV1":string, "error out"=w342:errorcluster)  [unwired: 13 in]
  n52 = call "GetSetProgramIntervalString.vi"("VISA resource name"=w340, "get/set"=w337, "Interval Number (Interval 0 is special case)"=w338, "error in"=w342) -> ("VISA resource name out"=w339:refnum<visa-resource-name>, "8800 Response"=→"8800 Get Response INTV2":string, "error out"=w341:errorcluster)  [unwired: 13 in]
  n53 = call "GetSetProgramDataString.vi"("VISA resource name"=w339, "get/set"=get_set."get", "8800 Program Name"=w354, "error in"=w341) -> ("VISA resource name out"=w327:refnum<visa-resource-name>, "Program get number of intervals"=→"Program get number of intervals":string, "error out"=w328:errorcluster)  [unwired: 9 in]
  n54 = call "GetThermAlarmAnalogInputChannelAvailability.vi"("error in"=w328, "ThermAlarm number"=w326, "VISA resource name"=w327) -> ("error out"=w324:errorcluster, "analog input channel available?"=→"analog input channel available?":i32, "VISA resource name out"=w323:refnum<visa-resource-name>)  [unwired: 6 in]
  n55 = call "GetIntervalTime.vi"("error in"=w324, "VISA resource name"=w323) -> ("error out"=w321:errorcluster, "Interval Time"=→"Interval Time":string, "VISA resource name out"=w320:refnum<visa-resource-name>)  [unwired: 7 in]
  n56 = call "GetInitialValue.vi"("error in"=w321, "Channel Number (1-4)"=w319, "VISA resource name"=w320) -> ("error out"=w316:errorcluster, "Current interval initial value"=→"Current interval initial value":sgl, "Current interval initial value string"=→"Current interval initial value string":string, "VISA resource name out"=w315:refnum<visa-resource-name>)  [unwired: 5 in]
  n57 = call "GetLanguageMode.vi"("error in"=w316, "VISA resource name"=w315) -> ("error out"=w309:errorcluster, "Language Mode Integer"=→"Language Mode Integer":i32, "Language Mode string"=→"Language Mode string":string, "VISA resource name out"=w308:refnum<visa-resource-name>)  [unwired: 6 in]
  n58 = call "GetSetLiveAux.vi"("VISA resource name"=w308, "get/set"=get_set."set", "Live Aux Number (1-8)"="Live Aux Number (1-8)", "State (o=off, 1=on)"="State (o=off, 1=on)", "error in"=w309) -> ("VISA resource name out"=w307:refnum<visa-resource-name>, "Live Aux State (0=off, 1=on)"=→"Live Aux State (0=off, 1=on)":i32, "Enabled? (0=disabled, 1=enabled)"=→"Enabled? (0=disabled, 1=enabled)":i32, "error out"=w310:errorcluster)  [unwired: 7 in]
  n59 = call "GetSetLiveAux.vi"("VISA resource name"=w307, "get/set"=get_set."get", "Live Aux Number (1-8)"="Live Aux Number (1-8)", "error in"=w310) -> ("VISA resource name out"=w299:refnum<visa-resource-name>, "Live Aux State (0=off, 1=on)"=→"Live Aux State (0=off, 1=on) 2":i32, "Enabled? (0=disabled, 1=enabled)"=→"Enabled? (0=disabled, 1=enabled) 2":i32, "error out"=w300:errorcluster)  [unwired: 8 in]
  n60 = call "GetSetLightStatus.vi"("error in"=w300, "Light status"=u8 0, "get/set"=w291, "VISA resource name"=w299) -> ("error out"=w298:errorcluster, "Light Status"=→"Light Status from Set":string, "VISA resource name out"=w297:refnum<visa-resource-name>)  [unwired: 5 in]
  n61 = call "GetSetLightStatus.vi"("error in"=w298, "get/set"=w290, "VISA resource name"=w297) -> ("error out"=w285:errorcluster, "Light Status"=→"Light Status from Get":string, "VISA resource name out"=w284:refnum<visa-resource-name>)  [unwired: 6 in]
  n62 = call "SetRunProgram.vi"("error in (no error)"=w285, "8800 Program Name (without .pgm extension)"="test", "VISA resource name"=w284) -> ("error out"=w280:errorcluster, "VISA resource name out"=w283:refnum<visa-resource-name>)  [unwired: 7 in]
  n63 = call "Time Delay2"("error in (no error)"=w280) -> ("error out"=w279:errorcluster)  [unwired: 10 in]
  n64 = call "SetHold.vi"("error in"=w279, "VISA resource name"=w283) -> ("error out"=w47:errorcluster, "VISA resource name out"=w46:refnum<visa-resource-name>)  [unwired: 7 in, 1 out]
  n65 = call "GetSetTimeLeft.vi"("VISA resource name"=w46, "get/set"=w43, "Time input cluster"=T9 {"Hours\n(0-99)"=3, "Minutes\n(0-5999)"=4, "Seconds\n(0-359999)"=5}, "error in"=w47) -> ("VISA resource name out"=w33:refnum<visa-resource-name>, "Time left string"=→"Time left string 1":string, "error out"=w34:errorcluster)  [unwired: 12 in, 1 out]
  n66 = call "GetSetTimeLeft.vi"("VISA resource name"=w33, "get/set"=w24, "error in"=w34) -> ("VISA resource name out"=w31:refnum<visa-resource-name>, "Time left string"=→"Time left string 2":string, "error out"=w32:errorcluster)  [unwired: 13 in, 1 out]
  n67 = call "GetSetTimeLeft.vi"("VISA resource name"=w31, "get/set"=w43, "Time input cluster"=T9 {"Hours\n(0-99)"=0, "Minutes\n(0-5999)"=4000, "Seconds\n(0-359999)"=10}, "error in"=w32) -> ("VISA resource name out"=w29:refnum<visa-resource-name>, "error out"=w30:errorcluster)  [unwired: 12 in, 2 out]
  n68 = call "GetSetTimeLeft.vi"("VISA resource name"=w29, "get/set"=w24, "error in"=w30) -> ("VISA resource name out"=w27:refnum<visa-resource-name>, "Time left string"=→"Time left string 3":string, "error out"=w28:errorcluster)  [unwired: 13 in, 1 out]
  n69 = call "GetSetTimeLeft.vi"("VISA resource name"=w27, "get/set"=w43, "Time input cluster"=T9 {"Hours\n(0-99)"=0, "Minutes\n(0-5999)"=0, "Seconds\n(0-359999)"=234}, "error in"=w28) -> ("VISA resource name out"=w35:refnum<visa-resource-name>, "error out"=w36:errorcluster)  [unwired: 12 in, 2 out]
  n70 = call "GetSetTimeLeft.vi"("VISA resource name"=w35, "get/set"=w24, "error in"=w36) -> ("VISA resource name out"=w44:refnum<visa-resource-name>, "Time left string"=→"Time left string 4":string, "Time left cluster"=w40:T2, "error out"=w45:errorcluster)  [unwired: 13 in]
  "Time left cluster" <- w40
  n71 = Unbundle By Name(w40) -> ("hours"=→"hours":i32, "minutes"=→"minutes":i32, "seconds"=→"seconds":i32)
  n72 = call "GetSetProgramLoopsLeft.vi"("error in"=w45, "Loops left"=u16 99, "get/set"=w291, "VISA resource name"=w44) -> ("error out"=w293:errorcluster, "Loops left?"=→"Loops left status":string, "VISA resource name out"=w292:refnum<visa-resource-name>)  [unwired: 5 in]
  n73 = call "GetSetProgramLoopsLeft.vi"("error in"=w293, "get/set"=w290, "VISA resource name"=w292) -> ("error out"=w278:errorcluster, "Loops left?"=→"Loops left?":string, "VISA resource name out"=w281:refnum<visa-resource-name>)  [unwired: 6 in]
  n74 = call "Time Delay3"("error in (no error)"=w278) -> ("error out"=w277:errorcluster)  [unwired: 10 in]
  n75 = call "SetRunManual.vi"("error in"=w277, "VISA resource name"=w281) -> ("error out"=w276:errorcluster, "VISA resource name out"=w282:refnum<visa-resource-name>)  [unwired: 7 in, 1 out]
  n76 = call "Time Delay4"("error in (no error)"=w276) -> ("error out"=w275:errorcluster)  [unwired: 10 in]
  n77 = call "SetStop.vi"("error in"=w275, "VISA resource name"=w282) -> ("error out"=w269:errorcluster, "VISA resource name out"=w268:refnum<visa-resource-name>)  [unwired: 8 in]
  n78 = call "GetSetAccessLevel.vi"("error in"=w269, "Access level"=u8 2, "get/set"=get_set."set", "VISA resource name"=w268) -> ("error out"=w274:errorcluster, "Access level response"=→"Access level response set":string, "VISA resource name out"=w273:refnum<visa-resource-name>)  [unwired: 5 in]
  n79 = call "GetSetAccessLevel.vi"("error in"=w274, "get/set"=get_set."get", "VISA resource name"=w273) -> ("error out"=w263:errorcluster, "Access level response"=→"Access level response get":string, "VISA resource name out"=w262:refnum<visa-resource-name>)  [unwired: 6 in]
  n80 = call "GetSetMatchInterval.vi"("error in"=w263, "Match interval"=u16 3, "get/set"=get_set."set", "VISA resource name"=w262) -> ("error out"=w265:errorcluster, "Service request interval"=→"Service request interval status":string, "VISA resource name out"=w264:refnum<visa-resource-name>)  [unwired: 5 in]
  n81 = call "GetSetMatchInterval.vi"("error in"=w265, "get/set"=get_set."get", "VISA resource name"=w264) -> ("error out"=w252:errorcluster, "Service request interval"=→"Service request interval":string, "VISA resource name out"=w253:refnum<visa-resource-name>)  [unwired: 6 in]
  n82 = call "GetSetServiceRequestEventMask.vi"("VISA resource name"=w253, "get/set"=get_set."set", "Mask bits"=u8 170, "error in"=w252) -> ("VISA resource name out"=w249:refnum<visa-resource-name>, "SRQ event mask string"=→"Service request event mask status":string, "error out"=w250:errorcluster)  [unwired: 7 in, 2 out]
  n83 = call "GetSetServiceRequestEventMask.vi"("VISA resource name"=w249, "get/set"=get_set."get", "error in"=w250) -> ("VISA resource name out"=w246:refnum<visa-resource-name>, "SRQ event mask string"=→"Service request event mask string":string, "SRQ event mask"=→"Service request event mask":i32, "SRQ event mask binary"=→"Service request event mask binary":string, "error out"=w245:errorcluster)  [unwired: 8 in]
  n84 = call "GetServiceRequestStatus.vi"("VISA resource name"=w246, "error in"=w245) -> ("VISA resource name out"=w243:refnum<visa-resource-name>, "Service request status string"=→"Service request status string":string, "Service request status"=→"Service request status":i32, "Binary String"=→"Service request binary string":string, "error out"=w242:errorcluster)  [unwired: 9 in]
  n85 = call "GetSetSetpoint.vi"("VISA resource name"=w243, "get/set"=get_set."set", "Channel Number (1-4)"=w235, "Setpoint"=-5.8, "error in"=w242) -> ("VISA resource name out"=w238:refnum<visa-resource-name>, "Setpoint string"=→"Setpoint status":string, "error out"=w237:errorcluster)  [unwired: 7 in, 1 out]
  n86 = call "GetSetSetpoint.vi"("VISA resource name"=w238, "get/set"=get_set."get", "Channel Number (1-4)"=w235, "error in"=w237) -> ("VISA resource name out"=w233:refnum<visa-resource-name>, "Setpoint"=→"Setpoint":dbl, "error out"=w232:errorcluster)  [unwired: 8 in, 1 out]
  n87 = call "GetSerialNumber.vi"("error in"=w232, "VISA resource name"=w233) -> ("error out"=w230:errorcluster, "Chamber serial number"=→"Chamber serial number":string, "VISA resource name out"=w229:refnum<visa-resource-name>)  [unwired: 7 in]
  n88 = call "SetResetScreen.vi"("error in (no error)"=w230, "VISA resource name"=w229) -> ("error out"=w227:errorcluster, "8800 response"=→"reset screen response":string, "VISA resource name out"=w226:refnum<visa-resource-name>)  [unwired: 7 in]
  n89 = call "GetStopCode.vi"("error in"=w227, "VISA resource name"=w226) -> ("error out"=w224:errorcluster, "Stop code"=→"Stop code":string, "VISA resource name out"=w222:refnum<visa-resource-name>)  [unwired: 7 in]
  n90 = call "GetSetRealTimeClock.vi"("VISA resource name"=w222, "get/set"=get_set."set", "Date/Time"=T12 {"Month"="4", "Day"="10", "Hour"="05", "Minute"="4"}, "error in"=w224) -> ("VISA resource name out"=w221:refnum<visa-resource-name>, "Real time clock"=→"Real time clock set result":string, "error out"=w223:errorcluster)  [unwired: 9 in]
  n91 = call "GetSetRealTimeClock.vi"("VISA resource name"=w221, "get/set"=get_set."get", "error in"=w223) -> ("VISA resource name out"=w215:refnum<visa-resource-name>, "Real time clock"=→"Real time clock":string, "error out"=w216:errorcluster)  [unwired: 10 in]
  n92 = call "SetResume.vi"("error in"=w216, "VISA resource name"=w215) -> ("error out"=w213:errorcluster, "Resume result"=→"Resume result":string, "VISA resource name out"=w212:refnum<visa-resource-name>)  [unwired: 7 in]
  n93 = call "GetRefrigPressures.vi"("error in"=w213, "Refrig system number (1-4)"=w211, "VISA resource name"=w212) -> ("error out"=w205:errorcluster, "Refrig system pressures"=→"Refrig system pressures":string, "VISA resource name out"=w204:refnum<visa-resource-name>)  [unwired: 6 in]
  n94 = call "GetRefrigSystemStatus.vi"("VISA resource name"=w204, "Refrigeration system number (1-4)"=w209, "error in"=w205) -> ("VISA resource name out"=w193:refnum<visa-resource-name>, "Refrigeration system status string"=→"Refrigeration system status string":string, "Refrigeration system status"=→"Refrigeration system status":i32, "Refrigeration system status binary string"=→"Refrigeration system status binary string":string, "error out"=w194:errorcluster)  [unwired: 8 in]
  n95 = call "GetSetPowerFailRecovery.vi"("VISA resource name"=w193, "get/set"=get_set."set", "Enabled?"=w199, "Time"=u16 15, "Power Recovery Mode"=w195, "error in"=w194) -> ("VISA resource name out"=w203:refnum<visa-resource-name>, "Power fail recovery response"=→"Power fail recovery set response":string, "error out"=w202:errorcluster)  [unwired: 11 in]
  n96 = call "GetSetPowerFailRecovery.vi"("VISA resource name"=w203, "get/set"=get_set."get", "error in"=w202) -> ("VISA resource name out"=w190:refnum<visa-resource-name>, "Power fail recovery response"=→"Power fail recovery response":string, "error out"=w192:errorcluster)  [unwired: 14 in]
  n97 = call "GetProcessVariable.vi"("error in"=w192, "Channel (1-140)"=u16 1, "VISA resource name"=w190) -> ("error out"=w187:errorcluster, "Process Variable"=→"Process Variable":string, "VISA resource name out"=w186:refnum<visa-resource-name>)  [unwired: 6 in]
  n98 = call "GetProgramTimeRemaining.vi"("error in"=w187, "VISA resource name"=w186) -> ("error out"=w184:errorcluster, "Program time remaining"=→"Program time remaining":string, "VISA resource name out"=w183:refnum<visa-resource-name>)  [unwired: 7 in]
  n99 = call "GetProgramTime.vi"("error in"=w184, "VISA resource name"=w183) -> ("error out"=w180:errorcluster, "Program time"=→"Program time":string, "VISA resource name out"=w178:refnum<visa-resource-name>)  [unwired: 7 in]
  n100 = disable-structure shown="Enabled" {
    disable-tunnel: w180 -> [w537 w542]
    disable-tunnel: [w536 w542] -> w179
    disable-tunnel: w178 -> [w535 w543]
    disable-tunnel: [w534 w543] -> w177
    frame Disabled {
      n101 = call "SetProgramDataString.vi"("VISA resource name"=w535, "get/set"=get_set."set", "8800 Program Name (without .pgm extension)"="montetest", "Number of intervals in program"=u16 9, "error in (no error)"=w537) -> ("VISA resource name out"=w534:refnum<visa-resource-name>, "8800 response"=→"8800 response":string, "error out"=w536:errorcluster)  [unwired: 8 in]
    }
    frame Enabled {
    }
  }
  n102 = call "SetProgramDataString.vi"("VISA resource name"=w177, "get/set"=get_set."get", "error in (no error)"=w179) -> ("VISA resource name out"=w173:refnum<visa-resource-name>, "8800 response"=→"8800 program":string, "error out"=w174:errorcluster)  [unwired: 10 in]
  n103 = call "GetSetParameterGroup.vi"("error in"=w174, "Parameter group number (1-4)"=u8 1, "get/set"=get_set."set", "VISA resource name"=w173) -> ("error out"=w175:errorcluster, "Parameter group response"=→"Parameter group response":string, "VISA resource name out"=w176:refnum<visa-resource-name>)  [unwired: 4 in]
  n104 = call "GetSetParameterGroup.vi"("error in"=w175, "get/set"=get_set."get", "VISA resource name"=w176) -> ("error out"=w167:errorcluster, "Parameter group response"=→"Parameter group":string, "VISA resource name out"=w166:refnum<visa-resource-name>)  [unwired: 5 in]
  n105 = call "GetProgramName.vi"("error in"=w167, "VISA resource name"=w166) -> ("error out"=w164:errorcluster, "Currently loaded program name response"=→"Currently loaded program name response":string, "VISA resource name out"=w162:refnum<visa-resource-name>)  [unwired: 7 in]
  n106 = call "GetSetParameterValues.vi"("VISA resource name"=w162, "get/set"=get_set."get", "Control channel number (1-4)"=w134, "Parameter group number (1-4)"=w133, "error in"=w164) -> ("VISA resource name out"=w161:refnum<visa-resource-name>, "Parameter values response"=w159:string, "error out"=w163:errorcluster)  [unwired: 12 in]
  "Parameter values response" <- w159
  n107 = Scan String For Tokens(6:w148, 9:w159) -> (1:w145:string, 2:w158:i32, 3:w157:string)  [unwired: 4 in, 1 out]
  n108 = Scan String For Tokens(6:w148, 8:w158, 9:w157) -> (1:w144:string, 2:w152:i32, 3:w156:string)  [unwired: 3 in, 1 out]
  n109 = Scan String For Tokens(6:w148, 8:w152, 9:w156) -> (1:w143:string, 2:w151:i32, 3:w155:string)  [unwired: 3 in, 1 out]
  n110 = Decimal String To Number(string=w143) -> (number=w127:i32)  [unwired: 2 in, 1 out]
  n111 = Scan String For Tokens(6:w148, 8:w151, 9:w155) -> (1:w142:string, 2:w150:i32, 3:w154:string)  [unwired: 3 in, 1 out]
  n112 = Decimal String To Number(string=w142) -> (number=w126:i32)  [unwired: 2 in, 1 out]
  n113 = Scan String For Tokens(6:w148, 8:w150, 9:w154) -> (1:w140:string, 2:w149:i32, 3:w153:string)  [unwired: 3 in, 1 out]
  n114 = Scan String For Tokens(6:w148, 8:w149, 9:w153) -> (1:w139:string)  [unwired: 3 in, 3 out]
  n115 = Scan From String(format string=w141, input string=w145) -> (output 1=w129:dbl)  [unwired: 3 in, 3 out]
  n116 = Scan From String(format string=w141, input string=w144) -> (output 1=w128:dbl)  [unwired: 3 in, 3 out]
  n117 = Scan From String(format string=w141, input string=w140) -> (output 1=w125:dbl)  [unwired: 3 in, 3 out]
  n118 = Scan From String(format string=w141, input string=w139) -> (output 1=w124:dbl)  [unwired: 3 in, 3 out]
  n119 = Bundle By Name(cluster=T19 {"Heat Gain"=0.0, "Heat IT"=0, "Heat Off"=0.0, "Cool Off"=0.0, "Cool Gain"=0.0, "Cool IT"=0} ("PTC operation"), "Heat Gain"=w129, "Cool Gain"=w128, "Heat IT"=w127, "Cool IT"=w126, "Heat Off"=w125, "Cool Off"=w124) -> (w130:T19)
  n120 = Bundle By Name(cluster=T20 {"Heat PB"=0.0, "Heat IT"=0, "Heat TL"=0.0, "Cool TL"=0.0, "Cool PB"=0.0, "Cool IT"=0} ("Non-PTC operation"), "Heat PB"=w129, "Cool PB"=w128, "Heat IT"=w127, "Cool IT"=w126, "Heat TL"=w125, "Cool TL"=w124) -> (w138:T20)
  n121 = call "GetSetParameterValues.vi"("VISA resource name"=w161, "get/set"=w135, "Control channel number (1-4)"=w134, "Parameter group number (1-4)"=w133, "Select Non-PTC(F) or PTC(T)"=FALSE, "error in"=w163, "Non-PTC operation"=w138) -> ("VISA resource name out"=w136:refnum<visa-resource-name>, "Parameter values response"=→"Parm response":string, "error out"=w137:errorcluster)  [unwired: 10 in]
  n122 = call "GetSetParameterValues.vi"("VISA resource name"=w136, "get/set"=w135, "Control channel number (1-4)"=w134, "Parameter group number (1-4)"=w133, "Select Non-PTC(F) or PTC(T)"=TRUE, "error in"=w137, "PTC operation"=w130) -> ("VISA resource name out"=w120:refnum<visa-resource-name>, "Parameter values response"=→"Parm response 2":string, "error out"=w121:errorcluster)  [unwired: 10 in]
  n123 = call "GetLowProcessAlarmLimit.vi"("error in"=w121, "Channel Number (1-4)"=w116, "VISA resource name"=w120) -> ("error out"=w118:errorcluster, "Low process alarm limit"=→"Low process alarm limit":string, "VISA resource name out"=w117:refnum<visa-resource-name>)  [unwired: 6 in]
  n124 = call "GetHighProcessAlarmLimit.vi"("error in"=w118, "Channel Number (1-4)"=w116, "VISA resource name"=w117) -> ("error out"=w108:errorcluster, "High process alarm limit"=→"High process alarm limit":string, "VISA resource name out"=w107:refnum<visa-resource-name>)  [unwired: 5 in]
  n125 = call "GetSetControllerOptions.vi"("error in"=w108, "Option (may be added for multiple)"=w106, "get/set"=get_set."set", "VISA resource name"=w107) -> ("error out"=w114:errorcluster, "Option response"=→"Option response set":string, "VISA resource name out"=w113:refnum<visa-resource-name>)  [unwired: 5 in]
  n126 = call "GetSetControllerOptions.vi"("error in"=w114, "get/set"=get_set."get", "VISA resource name"=w113) -> ("error out"=w104:errorcluster, "Option response"=→"Option response get":string, "VISA resource name out"=w103:refnum<visa-resource-name>)  [unwired: 6 in]
  n127 = call "GetNextInterval.vi"("error in"=w104, "VISA resource name"=w103) -> ("error out"=w100:errorcluster, "Next interval"=→"Next interval":i32, "VISA resource name out"=w99:refnum<visa-resource-name>)  [unwired: 6 in, 1 out]
  n128 = call "GetNumberOfLoops.vi"("error in"=w100, "VISA resource name"=w99) -> ("error out"=w95:errorcluster, "Number of loops"=→"Number of loops":i32, "Number of loops string"=→"Number of loops string":string, "VISA resource name out"=w96:refnum<visa-resource-name>)  [unwired: 6 in]
  n129 = call "GetSetControlledStopParms.vi"("error in"=w95, "Input parms"="Input parms", "get/set"=get_set."set", "VISA resource name"=w96) -> ("error out"=w94:errorcluster, "Controlled stop parms response"=→"Controlled stop parms response from set":string, "VISA resource name out"=w93:refnum<visa-resource-name>)  [unwired: 5 in]
  n130 = call "GetSetControlledStopParms.vi"("error in"=w94, "get/set"=get_set."get", "VISA resource name"=w93) -> ("error out"=w87:errorcluster, "Controlled stop parms response"=→"Controlled stop parms response":string, "VISA resource name out"=w88:refnum<visa-resource-name>)  [unwired: 6 in]
  n131 = call "GetOperatingMode.vi"("VISA resource name"=w88, "error in"=w87) -> ("VISA resource name out"=w82:refnum<visa-resource-name>, "Operating mode string"=→"Operating mode string":string, "Operating mode"=→"Operating mode":u8, "Operating mode binary"=→"Operating mode binary":string, "error out"=w83:errorcluster)  [unwired: 9 in]
  n132 = call "GetMonitorChannelValue.vi"("error in"=w83, "Channel number (1-24)"=1, "VISA resource name"=w82) -> ("error out"=w78:errorcluster, "Monitor channel value"=→"Monitor channel value":sgl, "Monitor Channel Value String"=→"Monitor Channel Value String":string, "VISA resource name out"=w77:refnum<visa-resource-name>)  [unwired: 5 in]
  n133 = call "GetSetManualRamp.vi"("VISA resource name"=w77, "get/set"=get_set."set", "Channel Number (1-4)"=w71, "Set manual ramp"=sgl 2.345 ("Manual ramp setting"), "error in"=w78) -> ("VISA resource name out"=w76:refnum<visa-resource-name>, "Manual ramp setting string"=→"Manual ramp setting status":string, "error out"=w75:errorcluster)  [unwired: 7 in, 1 out]
  n134 = call "GetSetManualRamp.vi"("VISA resource name"=w76, "get/set"=get_set."get", "Channel Number (1-4)"=w71, "error in"=w75) -> ("VISA resource name out"=w66:refnum<visa-resource-name>, "Manual ramp setting string"=→"Manual ramp setting string":string, "Get manual ramp setting"=→"Manual ramp setting":sgl, "error out"=w67:errorcluster)  [unwired: 8 in]
  n135 = call "SetWatchdogTimer.vi"("error in"=w67, "Watchdog timer seconds (0-600)"=i16 0, "VISA resource name"=w66) -> ("error out"=w63:errorcluster, "Reset watchdog timer result"=→"Reset watchdog timer result":string, "VISA resource name out"=w62:refnum<visa-resource-name>)  [unwired: 6 in]
  n136 = call "GetThermAlarmStatusFlags.vi"("VISA resource name"=w62, "error in"=w63) -> ("VISA resource name out"=w60:refnum<visa-resource-name>, "error out"=w61:errorcluster)  [unwired: 12 in, 4 out]
  n137 = call "GetThermAlarmAnalogInputValue.vi"("error in"=w61, "ThermAlarm number"=w55, "VISA resource name"=w60) -> ("error out"=w57:errorcluster, "ThermAlarm analog input value"=→"ThermAlarm analog input value":i32, "ThermAlarm analog input value string"=→"ThermAlarm analog input value string":string, "VISA resource name out"=w56:refnum<visa-resource-name>)  [unwired: 5 in]
  n138 = call "GetThermAlarmTemperature.vi"("error in"=w57, "ThermAlarm number"=w55, "VISA resource name"=w56) -> ("error out"=w52:errorcluster, "ThermAlarm temperature"=→"ThermAlarm temperature":i32, "ThermAlarm temperature string"=→"ThermAlarm temperature string":string, "VISA resource name out"=w51:refnum<visa-resource-name>)  [unwired: 5 in]
  n139 = call "GetThrottleReading.vi"("error in"=w52, "Channel Number (1-8)"=w50, "VISA resource name"=w51) -> ("error out"=w21:errorcluster, "Throttle reading"=→"Throttle reading":i8, "Throttle reading string"=→"Throttle reading string":string, "VISA resource name out"=w20:refnum<visa-resource-name>)  [unwired: 5 in]
  n140 = call "GetSetTemperatureScale.vi"("VISA resource name"=w20, "get/set"=get_set."set", "Temperature scale"=w17, "error in"=w21) -> ("VISA resource name out"=w22:refnum<visa-resource-name>, "Temperature scale string\n(0=Celsius; 1=Fahrenheit)"=→"Temperature scale result":string, "error out"=w23:errorcluster)  [unwired: 7 in, 2 out]
  n141 = call "GetSetTemperatureScale.vi"("VISA resource name"=w22, "get/set"=get_set."get", "error in"=w23) -> ("VISA resource name out"=w11:refnum<visa-resource-name>, "Temperature scale string\n(0=Celsius; 1=Fahrenheit)"=→"Temperature scale":string, "Temperature scale\n(0=Celsius; 1=Fahrenheit)"=→"Temperature scale\n(0=Celcius; 1=Fahrenheit)":u8, "Temperature scale text"=→"Temperature scale text":string, "error out"=w12:errorcluster)  [unwired: 8 in]
  n142 = call "GetSoftwareVersion.vi"("error in"=w12, "VISA resource name"=w11) -> ("error out"=w9:errorcluster, "Software version"=→"Software version":string, "VISA resource name out"=w10:refnum<visa-resource-name>)  [unwired: 7 in]
  n143 = call "Close.vi"("error in (no error)"=w9, "VISA resource name"=w10) -> ("error out"=→"error out":errorcluster)  [unwired: 9 in]
